vi "Launch Shape Dialog.vi"(8 "error in (no error)":errorcluster, 9 "Async?":bool, 10 "ShapeRef":refnum<data-value>, 11 "Editor Handler in":refnum<class "Image Editor Handler.lvclass">) -> (0 "error out":errorcluster, 3 "Editor Handler out":refnum<class "Image Editor Handler.lvclass">)   [LabVIEW 2015, in "LV Image Editor Framework.lvlib" / "Image Editor Handler.lvclass"]
uses:
  Image Editor Handler.lvclass
  Forms/Shape/Shape.lvclass
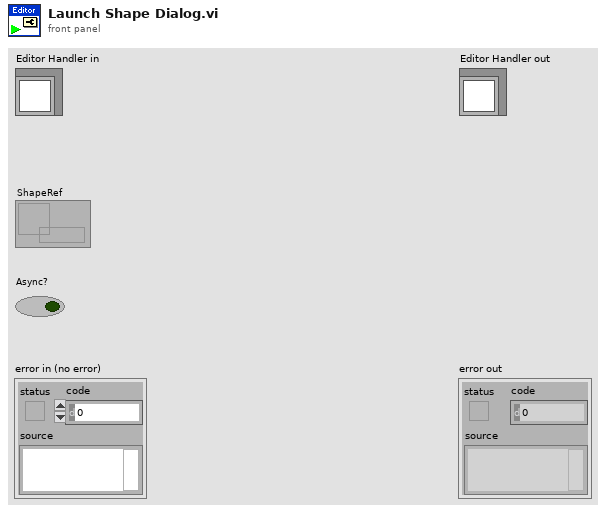
[diagram p1: front panel]
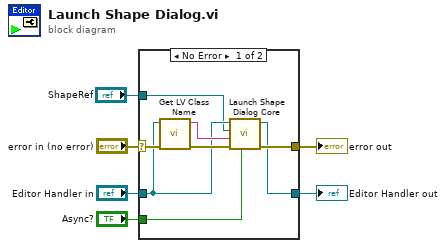
[diagram p0: block diagram]
diagram:
  n1 = case shown="No Error" "error in (no error)" {
    selector: "error in (no error)" -> [w14 w16]
    tunnel: [w9 w16] -> w5
    tunnel: [w8 w15] -> w3
    tunnel: "Editor Handler in" -> [w11 w15]
    tunnel: "Async?" -> [w7 _]
    tunnel: "ShapeRef" -> [w10 _]
    frame No Error {
      n2 = call <vilib>:"Get LV Class Name.vi"("error in (no error)"=w14, "object"=w11) -> ("error out"=w12:errorcluster, "class name"=w13:string)  [unwired: 8 in]
      n3 = call "Launch Shape Dialog Core.vi"("Async?"=w7, "error in (no error)"=w12, "class name"=w13, "ShapeRef"=w10, "Editor Handler in"=w11) -> ("error out"=w9:errorcluster, "Editor Handler out"=w8:refnum<class "Image Editor Handler.lvclass">)  [unwired: 5 in]
    }
    frame Error {
    }
  }
  "error out" <- w5
  "Editor Handler out" <- w3
